vi "read maps dynamically.vi"(8 "error in":errorcluster, 11 "Asynchronous Component Configuration In":refnum<class "asynchronous execution module configuration.lvclass">) -> (0 "error out":errorcluster, 2 "maps dynamically":bool, 3 "Asynchronous Component Configuration Out":refnum<class "asynchronous execution module configuration.lvclass">)   [LabVIEW 2013, in "asynchronous execution module configuration.lvclass"]
doc: "Provides an interface for determining if a runtime component associated with this configuration is capable of dynamically mapping to channels through <b>dynamic mapping.vi</b>."
uses:
  asynchronous execution module configuration.lvclass
  asynchronous execution module configuration.lvclass/asynchronous execution module configuration.ctl
  <vilib>/NI/Tag Bus Module Framework/module configuration/TBM module configuration.lvclass
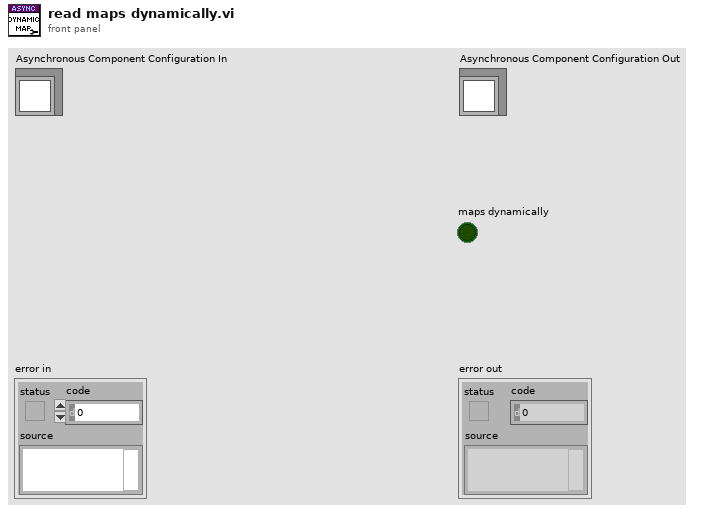
[diagram p1: front panel]
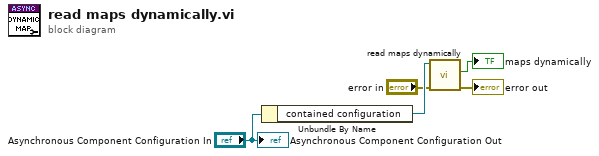
[diagram p0: block diagram]
diagram:
  n1 = Unbundle By Name("Asynchronous Component Configuration In") -> ("contained configuration"=w4:refnum<class "TBM module configuration.lvclass">)
  n2 = call-dynamic "read maps dynamically.vi"("error in"="error in", "module configuration in"=w4) -> ("error out"=→"error out":errorcluster, "maps dynamically"=→"maps dynamically":bool)  [unwired: 7 in, 1 out]
  "Asynchronous Component Configuration Out" <- "Asynchronous Component Configuration In"
